vi "Destroy.vi"(8 "error in (no error)":errorcluster, 11 "Event Registration Refnum":refnum<event-registration>) -> (0 "error out":errorcluster)   [LabVIEW 2020, in "WebServiceImporter.lvlib" / "Main Panel.lvlib" / "Finish.lvlib" / "Events.lvlib"]
uses:
  <vilib>/Platform/WebService/Main Panel/Pages/Finish/Events/Events.lvlib
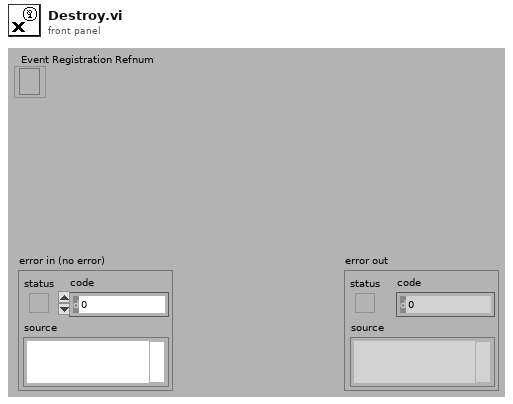
[diagram p1: front panel]
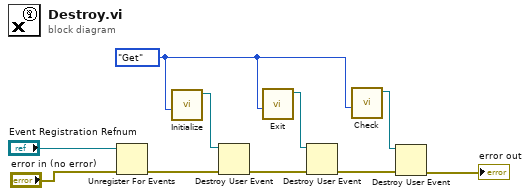
[diagram p0: block diagram]
diagram:
  w8 = enum16{"Get", "Set"}."Get" ("Operation")
  n1 = Unregister For Events(event registration refnum="Event Registration Refnum", error in="error in (no error)") -> (error out=w7:errorcluster)
  n2 = call <vilib>:"Initialize.vi"("Operation"=w8) -> ("user event (out)"=w6:refnum<user-event>)  [unwired: 10 in]
  n3 = Destroy User Event(user event=w6, error in=w7) -> (error out=w5:errorcluster)
  n4 = call <vilib>:"Exit.vi"("Operation"=w8) -> ("user event (out)"=w4:refnum<user-event>)  [unwired: 9 in, 1 out]
  n5 = Destroy User Event(user event=w4, error in=w5) -> (error out=w3:errorcluster)
  n6 = call <vilib>:"Check.vi"("Operation"=w8) -> ("user event (out)"=w2:refnum<user-event>)  [unwired: 9 in, 1 out]
  n7 = Destroy User Event(user event=w2, error in=w3) -> (error out=→"error out":errorcluster)
